vi "AlphaBetaToABC_src.vi"   [LabVIEW 2017]
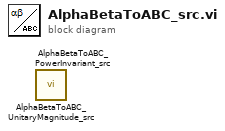
[diagram p0: block diagram]
diagram:
  n1 = call "AlphaBetaToABC_UnitaryMagnitude_src.vi"() -> ()  [unwired: 13 in, 3 out]
  n2 = call "AlphaBetaToABC_PowerInvariant_src.vi"() -> ()  [unwired: 13 in, 3 out]
